vi "get SPAN active components indices.vi"(8 "error in (no error)":errorcluster caption="Fehler (Eingang, kein Fehler)", 10 "SPAN Idx":i32, 11 "SpanInletClusterArray in":T1[](array[typedef]) {"zusätzliche Zeitdauer Erster Punkt" min=30 step=1 format="%#_5g"; "Zeitdauer Stufen" format="%#_5g"; "Max Fehler" format="%#_5g"; "Anzahl Stufen" format="%#_5g"; "Komponenten"."Komponente 5"."Komponente:" items=["NO (350,3000) LP 191C", "NO2 (150) LP 191C (1of2)", "NO2 (2000) LP 191C (2of2)", "N2O (300) LP 191C (1of2)", "NH3 (300) LP 191C (1of2)", "NH3 (900,3000) LP 191C (2of2)", "HNCO (400) 191C", "H2O% (30) LP 191C", "Formaldehyde (70,500) LP 191C", "CO2 low% (4) LP 191C (2of2)", "CO2% (20) LP 191C (1of2)", "CO (700) LP 191C (1of3)", "CO% (1) LP 191C (2of3)", "Propylene (1000) LP 191C", "Aromatic HC C7 (500) LP 191C", "Ethylene (1000) LP 191C", "CH4 (250) LP 191C (1of2)", "CH4 (5000) LP 191C (2of2)", "Ethane (1000) LP 191C", "Acetylene (1000) LP 191C", "HNO2 (20) 191C", "MeOH (1000) 191C", "CO% (10) LP 191C (3of3)", "Formic Acid (100) 191C", "SO2 (500) LP 191C", "Acetaldehyde (1000) LP 191C", "COS (100) LP 191C", "1,3 butadiene (100) LP 191C", "Oil as Octane (200) LP 191C", "N2O (1000) LP 191C (2of2)", "Propane (200) LP 191C", "NO2 autorange (2000)", "CO autorange (100000)", "CH4 autorange (5000)", "NH3 autorange (3000)", "Temp. Gascell", "Pressure Gascell", "sBeam@2500"]; "Komponenten"."Komponente 5"."Konzentration IST" format="%#.4f"; "Komponenten"."Komponente 5"."Genauigkeit" format="%#.1f"; "Komponenten"."Komponente 4"."Komponente:" items=["NO (350,3000) LP 191C", "NO2 (150) LP 191C (1of2)", "NO2 (2000) LP 191C (2of2)", "N2O (300) LP 191C (1of2)", "NH3 (300) LP 191C (1of2)", "NH3 (900,3000) LP 191C (2of2)", "HNCO (400) 191C", "H2O% (30) LP 191C", "Formaldehyde (70,500) LP 191C", "CO2 low% (4) LP 191C (2of2)", "CO2% (20) LP 191C (1of2)", "CO (700) LP 191C (1of3)", "CO% (1) LP 191C (2of3)", "Propylene (1000) LP 191C", "Aromatic HC C7 (500) LP 191C", "Ethylene (1000) LP 191C", "CH4 (250) LP 191C (1of2)", "CH4 (5000) LP 191C (2of2)", "Ethane (1000) LP 191C", "Acetylene (1000) LP 191C", "HNO2 (20) 191C", "MeOH (1000) 191C", "CO% (10) LP 191C (3of3)", "Formic Acid (100) 191C", "SO2 (500) LP 191C", "Acetaldehyde (1000) LP 191C", "COS (100) LP 191C", "1,3 butadiene (100) LP 191C", "Oil as Octane (200) LP 191C", "N2O (1000) LP 191C (2of2)", "Propane (200) LP 191C", "NO2 autorange (2000)", "CO autorange (100000)", "CH4 autorange (5000)", "NH3 autorange (3000)", "Temp. Gascell", "Pressure Gascell", "sBeam@2500"]; "Komponenten"."Komponente 4"."Konzentration IST" format="%#.4f"; "Komponenten"."Komponente 4"."Genauigkeit" format="%#.1f"; "Komponenten"."Komponente 3"."Komponente:" items=["NO (350,3000) LP 191C", "NO2 (150) LP 191C (1of2)", "NO2 (2000) LP 191C (2of2)", "N2O (300) LP 191C (1of2)", "NH3 (300) LP 191C (1of2)", "NH3 (900,3000) LP 191C (2of2)", "HNCO (400) 191C", "H2O% (30) LP 191C", "Formaldehyde (70,500) LP 191C", "CO2 low% (4) LP 191C (2of2)", "CO2% (20) LP 191C (1of2)", "CO (700) LP 191C (1of3)", "CO% (1) LP 191C (2of3)", "Propylene (1000) LP 191C", "Aromatic HC C7 (500) LP 191C", "Ethylene (1000) LP 191C", "CH4 (250) LP 191C (1of2)", "CH4 (5000) LP 191C (2of2)", "Ethane (1000) LP 191C", "Acetylene (1000) LP 191C", "HNO2 (20) 191C", "MeOH (1000) 191C", "CO% (10) LP 191C (3of3)", "Formic Acid (100) 191C", "SO2 (500) LP 191C", "Acetaldehyde (1000) LP 191C", "COS (100) LP 191C", "1,3 butadiene (100) LP 191C", "Oil as Octane (200) LP 191C", "N2O (1000) LP 191C (2of2)", "Propane (200) LP 191C", "NO2 autorange (2000)", "CO autorange (100000)", "CH4 autorange (5000)", "NH3 autorange (3000)", "Temp. Gascell", "Pressure Gascell", "sBeam@2500"]; "Komponenten"."Komponente 3"."Konzentration IST" format="%#.4f"; "Komponenten"."Komponente 3"."Genauigkeit" format="%#.1f"; "Komponenten"."Komponente 2"."Komponente:" items=["NO (350,3000) LP 191C", "NO2 (150) LP 191C (1of2)", "NO2 (2000) LP 191C (2of2)", "N2O (300) LP 191C (1of2)", "NH3 (300) LP 191C (1of2)", "NH3 (900,3000) LP 191C (2of2)", "HNCO (400) 191C", "H2O% (30) LP 191C", "Formaldehyde (70,500) LP 191C", "CO2 low% (4) LP 191C (2of2)", "CO2% (20) LP 191C (1of2)", "CO (700) LP 191C (1of3)", "CO% (1) LP 191C (2of3)", "Propylene (1000) LP 191C", "Aromatic HC C7 (500) LP 191C", "Ethylene (1000) LP 191C", "CH4 (250) LP 191C (1of2)", "CH4 (5000) LP 191C (2of2)", "Ethane (1000) LP 191C", "Acetylene (1000) LP 191C", "HNO2 (20) 191C", "MeOH (1000) 191C", "CO% (10) LP 191C (3of3)", "Formic Acid (100) 191C", "SO2 (500) LP 191C", "Acetaldehyde (1000) LP 191C", "COS (100) LP 191C", "1,3 butadiene (100) LP 191C", "Oil as Octane (200) LP 191C", "N2O (1000) LP 191C (2of2)", "Propane (200) LP 191C", "NO2 autorange (2000)", "CO autorange (100000)", "CH4 autorange (5000)", "NH3 autorange (3000)", "Temp. Gascell", "Pressure Gascell", "sBeam@2500"]; "Komponenten"."Komponente 2"."Konzentration IST" format="%#.4f"; "Komponenten"."Komponente 2"."Genauigkeit" format="%#.1f"; "Komponenten"."Komponente 1"."Komponente:" items=["NO (350,3000) LP 191C", "NO2 (150) LP 191C (1of2)", "NO2 (2000) LP 191C (2of2)", "N2O (300) LP 191C (1of2)", "NH3 (300) LP 191C (1of2)", "NH3 (900,3000) LP 191C (2of2)", "HNCO (400) 191C", "H2O% (30) LP 191C", "Formaldehyde (70,500) LP 191C", "CO2 low% (4) LP 191C (2of2)", "CO2% (20) LP 191C (1of2)", "CO (700) LP 191C (1of3)", "CO% (1) LP 191C (2of3)", "Propylene (1000) LP 191C", "Aromatic HC C7 (500) LP 191C", "Ethylene (1000) LP 191C", "CH4 (250) LP 191C (1of2)", "CH4 (5000) LP 191C (2of2)", "Ethane (1000) LP 191C", "Acetylene (1000) LP 191C", "HNO2 (20) 191C", "MeOH (1000) 191C", "CO% (10) LP 191C (3of3)", "Formic Acid (100) 191C", "SO2 (500) LP 191C", "Acetaldehyde (1000) LP 191C", "COS (100) LP 191C", "1,3 butadiene (100) LP 191C", "Oil as Octane (200) LP 191C", "N2O (1000) LP 191C (2of2)", "Propane (200) LP 191C", "NO2 autorange (2000)", "CO autorange (100000)", "CH4 autorange (5000)", "NH3 autorange (3000)", "Temp. Gascell", "Pressure Gascell", "sBeam@2500"]; "Komponenten"."Komponente 1"."Konzentration IST" format="%#.4f"; "Komponenten"."Komponente 1"."Genauigkeit" format="%#.1f"; "Ablaufdatum" format="%<%d.%m.%Y>T"; "Gasflasche" items=["----"=10000, "IAG NH3 3000"=0, "IAG NH3 200"=1, "IAG NH3 2000"=2, "IAG MG"=3, "IAG O2"=4]}) -> (0 "error out":errorcluster caption="Fehler (Ausgang)", 1 "aktive Komponenten Indices":i32[](array[numeric]), 2 "SPAN Idx out":i32, 3 "SpanInletClusterArray out":T1[](array[typedef]) {"zusätzliche Zeitdauer Erster Punkt" min=30 step=1 format="%#_5g"; "Zeitdauer Stufen" format="%#_5g"; "Max Fehler" format="%#_5g"; "Anzahl Stufen" format="%#_5g"; "Komponenten"."Komponente 5"."Komponente:" items=["NO (350,3000) LP 191C", "NO2 (150) LP 191C (1of2)", "NO2 (2000) LP 191C (2of2)", "N2O (300) LP 191C (1of2)", "NH3 (300) LP 191C (1of2)", "NH3 (900,3000) LP 191C (2of2)", "HNCO (400) 191C", "H2O% (30) LP 191C", "Formaldehyde (70,500) LP 191C", "CO2 low% (4) LP 191C (2of2)", "CO2% (20) LP 191C (1of2)", "CO (700) LP 191C (1of3)", "CO% (1) LP 191C (2of3)", "Propylene (1000) LP 191C", "Aromatic HC C7 (500) LP 191C", "Ethylene (1000) LP 191C", "CH4 (250) LP 191C (1of2)", "CH4 (5000) LP 191C (2of2)", "Ethane (1000) LP 191C", "Acetylene (1000) LP 191C", "HNO2 (20) 191C", "MeOH (1000) 191C", "CO% (10) LP 191C (3of3)", "Formic Acid (100) 191C", "SO2 (500) LP 191C", "Acetaldehyde (1000) LP 191C", "COS (100) LP 191C", "1,3 butadiene (100) LP 191C", "Oil as Octane (200) LP 191C", "N2O (1000) LP 191C (2of2)", "Propane (200) LP 191C", "NO2 autorange (2000)", "CO autorange (100000)", "CH4 autorange (5000)", "NH3 autorange (3000)", "Temp. Gascell", "Pressure Gascell", "sBeam@2500"]; "Komponenten"."Komponente 5"."Konzentration IST" format="%#.4f"; "Komponenten"."Komponente 5"."Genauigkeit" format="%#.1f"; "Komponenten"."Komponente 4"."Komponente:" items=["NO (350,3000) LP 191C", "NO2 (150) LP 191C (1of2)", "NO2 (2000) LP 191C (2of2)", "N2O (300) LP 191C (1of2)", "NH3 (300) LP 191C (1of2)", "NH3 (900,3000) LP 191C (2of2)", "HNCO (400) 191C", "H2O% (30) LP 191C", "Formaldehyde (70,500) LP 191C", "CO2 low% (4) LP 191C (2of2)", "CO2% (20) LP 191C (1of2)", "CO (700) LP 191C (1of3)", "CO% (1) LP 191C (2of3)", "Propylene (1000) LP 191C", "Aromatic HC C7 (500) LP 191C", "Ethylene (1000) LP 191C", "CH4 (250) LP 191C (1of2)", "CH4 (5000) LP 191C (2of2)", "Ethane (1000) LP 191C", "Acetylene (1000) LP 191C", "HNO2 (20) 191C", "MeOH (1000) 191C", "CO% (10) LP 191C (3of3)", "Formic Acid (100) 191C", "SO2 (500) LP 191C", "Acetaldehyde (1000) LP 191C", "COS (100) LP 191C", "1,3 butadiene (100) LP 191C", "Oil as Octane (200) LP 191C", "N2O (1000) LP 191C (2of2)", "Propane (200) LP 191C", "NO2 autorange (2000)", "CO autorange (100000)", "CH4 autorange (5000)", "NH3 autorange (3000)", "Temp. Gascell", "Pressure Gascell", "sBeam@2500"]; "Komponenten"."Komponente 4"."Konzentration IST" format="%#.4f"; "Komponenten"."Komponente 4"."Genauigkeit" format="%#.1f"; "Komponenten"."Komponente 3"."Komponente:" items=["NO (350,3000) LP 191C", "NO2 (150) LP 191C (1of2)", "NO2 (2000) LP 191C (2of2)", "N2O (300) LP 191C (1of2)", "NH3 (300) LP 191C (1of2)", "NH3 (900,3000) LP 191C (2of2)", "HNCO (400) 191C", "H2O% (30) LP 191C", "Formaldehyde (70,500) LP 191C", "CO2 low% (4) LP 191C (2of2)", "CO2% (20) LP 191C (1of2)", "CO (700) LP 191C (1of3)", "CO% (1) LP 191C (2of3)", "Propylene (1000) LP 191C", "Aromatic HC C7 (500) LP 191C", "Ethylene (1000) LP 191C", "CH4 (250) LP 191C (1of2)", "CH4 (5000) LP 191C (2of2)", "Ethane (1000) LP 191C", "Acetylene (1000) LP 191C", "HNO2 (20) 191C", "MeOH (1000) 191C", "CO% (10) LP 191C (3of3)", "Formic Acid (100) 191C", "SO2 (500) LP 191C", "Acetaldehyde (1000) LP 191C", "COS (100) LP 191C", "1,3 butadiene (100) LP 191C", "Oil as Octane (200) LP 191C", "N2O (1000) LP 191C (2of2)", "Propane (200) LP 191C", "NO2 autorange (2000)", "CO autorange (100000)", "CH4 autorange (5000)", "NH3 autorange (3000)", "Temp. Gascell", "Pressure Gascell", "sBeam@2500"]; "Komponenten"."Komponente 3"."Konzentration IST" format="%#.4f"; "Komponenten"."Komponente 3"."Genauigkeit" format="%#.1f"; "Komponenten"."Komponente 2"."Komponente:" items=["NO (350,3000) LP 191C", "NO2 (150) LP 191C (1of2)", "NO2 (2000) LP 191C (2of2)", "N2O (300) LP 191C (1of2)", "NH3 (300) LP 191C (1of2)", "NH3 (900,3000) LP 191C (2of2)", "HNCO (400) 191C", "H2O% (30) LP 191C", "Formaldehyde (70,500) LP 191C", "CO2 low% (4) LP 191C (2of2)", "CO2% (20) LP 191C (1of2)", "CO (700) LP 191C (1of3)", "CO% (1) LP 191C (2of3)", "Propylene (1000) LP 191C", "Aromatic HC C7 (500) LP 191C", "Ethylene (1000) LP 191C", "CH4 (250) LP 191C (1of2)", "CH4 (5000) LP 191C (2of2)", "Ethane (1000) LP 191C", "Acetylene (1000) LP 191C", "HNO2 (20) 191C", "MeOH (1000) 191C", "CO% (10) LP 191C (3of3)", "Formic Acid (100) 191C", "SO2 (500) LP 191C", "Acetaldehyde (1000) LP 191C", "COS (100) LP 191C", "1,3 butadiene (100) LP 191C", "Oil as Octane (200) LP 191C", "N2O (1000) LP 191C (2of2)", "Propane (200) LP 191C", "NO2 autorange (2000)", "CO autorange (100000)", "CH4 autorange (5000)", "NH3 autorange (3000)", "Temp. Gascell", "Pressure Gascell", "sBeam@2500"]; "Komponenten"."Komponente 2"."Konzentration IST" format="%#.4f"; "Komponenten"."Komponente 2"."Genauigkeit" format="%#.1f"; "Komponenten"."Komponente 1"."Komponente:" items=["NO (350,3000) LP 191C", "NO2 (150) LP 191C (1of2)", "NO2 (2000) LP 191C (2of2)", "N2O (300) LP 191C (1of2)", "NH3 (300) LP 191C (1of2)", "NH3 (900,3000) LP 191C (2of2)", "HNCO (400) 191C", "H2O% (30) LP 191C", "Formaldehyde (70,500) LP 191C", "CO2 low% (4) LP 191C (2of2)", "CO2% (20) LP 191C (1of2)", "CO (700) LP 191C (1of3)", "CO% (1) LP 191C (2of3)", "Propylene (1000) LP 191C", "Aromatic HC C7 (500) LP 191C", "Ethylene (1000) LP 191C", "CH4 (250) LP 191C (1of2)", "CH4 (5000) LP 191C (2of2)", "Ethane (1000) LP 191C", "Acetylene (1000) LP 191C", "HNO2 (20) 191C", "MeOH (1000) 191C", "CO% (10) LP 191C (3of3)", "Formic Acid (100) 191C", "SO2 (500) LP 191C", "Acetaldehyde (1000) LP 191C", "COS (100) LP 191C", "1,3 butadiene (100) LP 191C", "Oil as Octane (200) LP 191C", "N2O (1000) LP 191C (2of2)", "Propane (200) LP 191C", "NO2 autorange (2000)", "CO autorange (100000)", "CH4 autorange (5000)", "NH3 autorange (3000)", "Temp. Gascell", "Pressure Gascell", "sBeam@2500"]; "Komponenten"."Komponente 1"."Konzentration IST" format="%#.4f"; "Komponenten"."Komponente 1"."Genauigkeit" format="%#.1f"; "Ablaufdatum" format="%<%d.%m.%Y>T"; "Gasflasche" items=["----"=10000, "IAG NH3 3000"=0, "IAG NH3 200"=1, "IAG NH3 2000"=2, "IAG MG"=3, "IAG O2"=4]}, 4 "Anzahl aktive Komponenten":i32)   [LabVIEW 2020, in "Linearisierung v2.lvlib" / "SpanEinstellungen.lvlib"]
uses:
  SpanEinstellungen.lvlib
  SpanInletCluster.ctl
  Seiten/System Einstellungen V2/Konfig Gasflasche.ctl
  Seiten/System Einstellungen V2/Analysatoren.ctl
  Seiten/System Einstellungen V2/Gasflasche Auswahl.ctl
  Komponentencluster mit Formel.ctl
  Komponentenauswahl mit Formel.ctl
  Visualisierungs Elemente/String - Eingabefeld.ctl
  Einheit.ctl
  Seiten/System Einstellungen V2/Traegergas.ctl
  Seiten/System Einstellungen V2/System Einstellungen V2.lvlib
panel:
  out "aktive Komponenten":u16[](array[numeric])
  # "sec"
  # "%"
  # "sec"
  # "Komponente"
  # "Formel"
  # "Konzentration"
  # "Einheit"
  # "Genauigkeit [%]"
  # "sec"
  # "%"
  # "sec"
  # "Komponente"
  # "Formel"
  # "Konzentration"
  # "Einheit"
  # "Genauigkeit [%]"
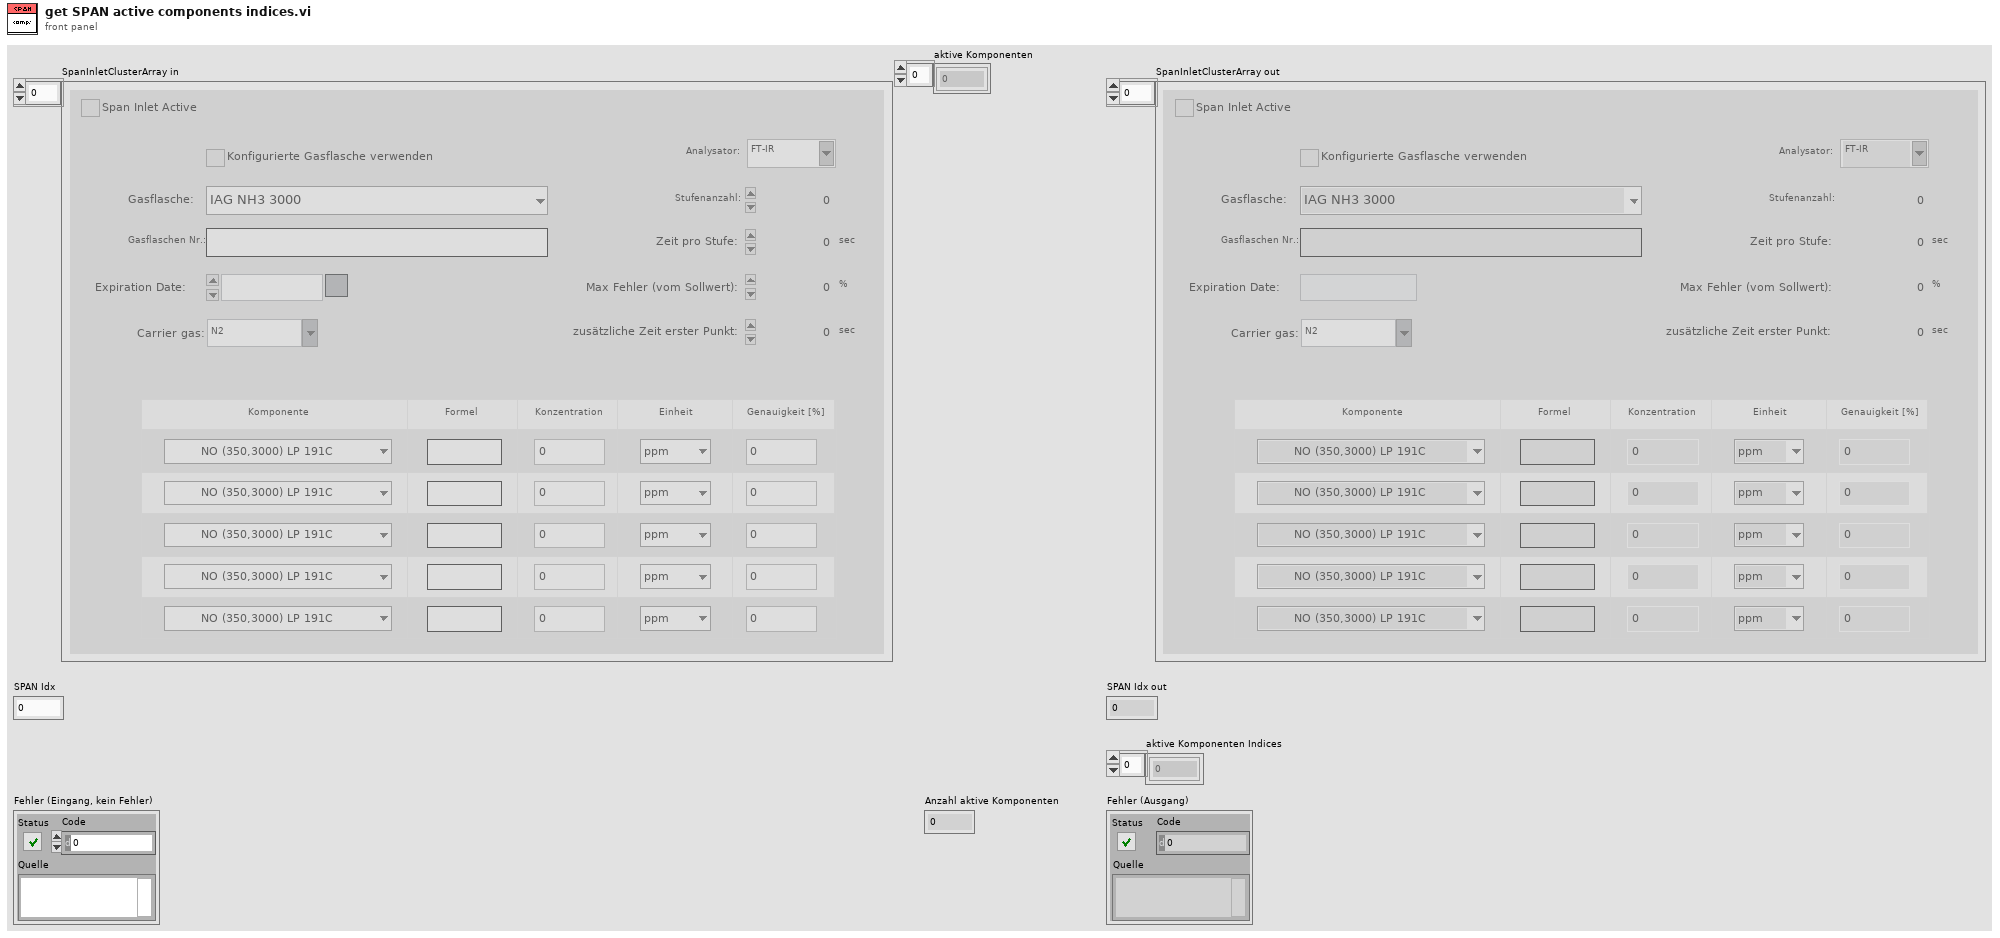
[diagram p1: front panel]
types:
  T1 = typedef "Linearisierung v2.lvlib/SpanEinstellungen.lvlib/SpanInletCluster.ctl" = cluster{"Span Inlet Active":T2, "Analysator":T3, "Konfig Gasflasche":T2, "Gasflasche":T4, "Gasflaschen Nr.:":string, "Ablaufdatum":timestamp, "Komponenten":T5, "Zeitdauer Stufen":sgl, "Max Fehler":sgl, "Anzahl Stufen":sgl, "Trägergas":T9, "zusätzliche Zeitdauer Erster Punkt":sgl}
  T2 = typedef "System Einstellungen V2.lvlib/Konfig Gasflasche.ctl" = bool
  T3 = typedef "System Einstellungen V2.lvlib/Analysatoren.ctl" = string
  T4 = typedef "System Einstellungen V2.lvlib/Gasflasche Auswahl.ctl" = u16
  T5 = typedef "Linearisierung v2.lvlib/SpanEinstellungen.lvlib/Komponentencluster mit Formel.ctl" = cluster{"Komponente 1":T6, "Komponente 2":T6, "Komponente 3":T6, "Komponente 4":T6, "Komponente 5":T6}
  T6 = typedef "Linearisierung v2.lvlib/SpanEinstellungen.lvlib/Komponentenauswahl mit Formel.ctl" = cluster{"Komponente:":u16, "Summenformel":T7, "Konzentration IST":dbl, "Einheit":T8, "Genauigkeit":dbl}
  T7 = typedef "String - Eingabefeld.ctl" = string
  T8 = typedef "Linearisierung v2.lvlib/SpanEinstellungen.lvlib/Einheit.ctl" = enum16{"ppm", "%"}
  T9 = typedef "System Einstellungen V2.lvlib/Traegergas.ctl" = string
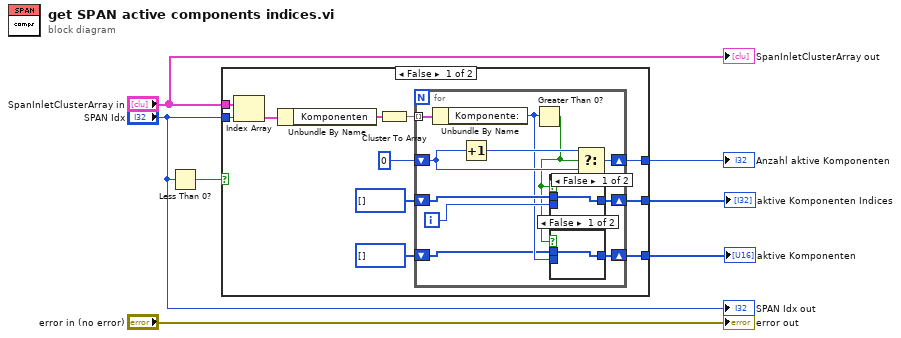
[diagram p0: block diagram]
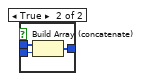
[diagram p2: hidden frame]
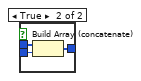
[diagram p3: hidden frame]
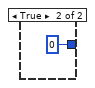
[diagram p4: hidden frame]
diagram:
  n1 = Less Than 0?(x="SPAN Idx") -> (x < 0?=w4:bool)
  n2 = case shown="False" w4 {
    tunnel: "SpanInletClusterArray in" -> [w18 _]
    tunnel: [w13 0] -> w6
    tunnel: "SPAN Idx" -> [w12 _]
    tunnel: [w11 _] -> w2
    tunnel: [w9 _] -> w1
    frame False {
      n3 = Index Array(array=w18, index=w12) -> (element=w17:T1)
      n4 = Unbundle By Name(w17) -> ("Komponenten"=w16:T5)
      n5 = Cluster To Array(cluster=w16) -> (array=w15:T6[])
      n6 = for {
        tunnel: w15 -> [w29] mode=indexing
        shift-right: [w28] -> w13
        shift-left: 0 -> [w26]
        shift-right: [w24] -> w11
        shift-left: i32[] [] -> [w23]
        shift-right: [w21] -> w9
        shift-left: u16[] [] -> [w20]
        i -> [w25]
        n7 = Unbundle By Name(w29) -> ("Komponente:"=w22:u16)
        n8 = Increment(x=w26) -> (x+1=w27:i32)
        n9 = Greater Than 0?(x=w22) -> (x > 0?=w19:bool)
        n10 = case shown="False" w19 {
          tunnel: w25 -> [_ w37]
          tunnel: [w34 w36] -> w24
          tunnel: w23 -> [w34 w35]
          frame False {
          }
          frame True {
            n11 = Build Array (concatenate)(w35, w37) -> (w36:i32[])
          }
        }
        n12 = case shown="False" w19 {
          tunnel: w22 -> [_ w33]
          tunnel: [w30 w32] -> w21
          tunnel: w20 -> [w30 w31]
          frame False {
          }
          frame True {
            n13 = Build Array (concatenate)(w31, w33) -> (w32:u16[])
          }
        }
        n14 = Select(t=w27, s=w19, f=w26) -> (s? t:f=w28:i32)
      }
    }
    frame True {
    }
  }
  "Anzahl aktive Komponenten" <- w6
  "aktive Komponenten Indices" <- w2
  "aktive Komponenten" <- w1
  "SPAN Idx out" <- "SPAN Idx"
  "SpanInletClusterArray out" <- "SpanInletClusterArray in"
  "error out" <- "error in (no error)"
